vi "MuxReset.vi"(8 "error in (no error)":errorcluster, 11 "GPIBSwitching in":refnum<class "GPIBSwitching.lvclass">) -> (0 "error out":errorcluster, 3 "GPIBSwitching out":refnum<class "GPIBSwitching.lvclass">)   [LabVIEW 2018, in "GPIBSwitching.lvclass"]
uses:
  GPIBSwitching.lvclass
  C:/ProbeTestSoftware2019/itk-strip-sensor-qc/InstrControl/InstrControl.lvclass
  MUX_CommandsGlobal.vi
  InstrControl.lvclass
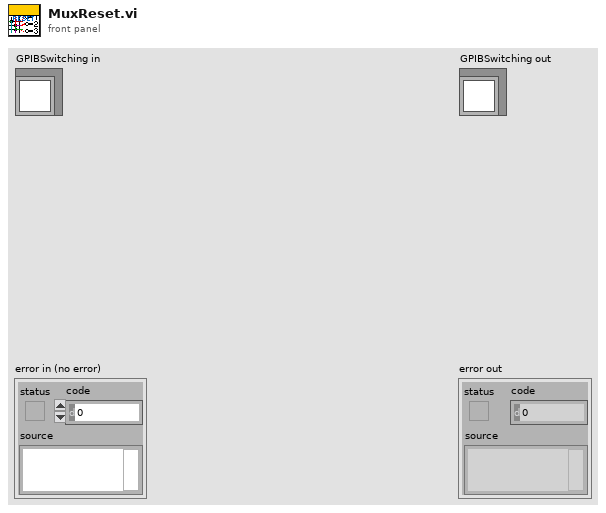
[diagram p1: front panel]
types:
  T1 = cluster{"Mux1 address":string, "Mux2 address":string, "Instrument name":string, "Instrument type":u16, "Command \"MUX Reset\"":string, "Command \"Select MUX Channel\"":string}
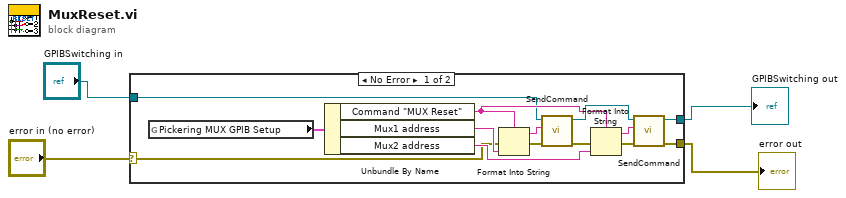
[diagram p0: block diagram]
diagram:
  n1 = case shown="No Error" "error in (no error)" {
    selector: "error in (no error)" -> [w5 w20]
    tunnel: [w13 w20] -> w3
    tunnel: [w17 w19] -> w4
    tunnel: "GPIBSwitching in" -> [w6 w19]
    frame No Error {
      n2 = global read "MUX_CommandsGlobal.vi" "Pickering MUX GPIB Setup"() -> (w12:T1)
      n3 = Unbundle By Name(w12) -> ("Command \"MUX Reset\""=w11:string, "Mux1 address"=w10:string, "Mux2 address"=w9:string)
      n4 = Format Into String(format string=w11, error in=w5, w10) -> (resulting string=w8:string, error out=w16:errorcluster)  [unwired: 1 in]
      n5 = call "SendCommand.vi"("error in (no error)"=w16, "Command string"=w8, "InstControl in"=w6) -> ("error out"=w15:errorcluster, "InstControl out"=w18:refnum<class "GPIBSwitching.lvclass">)  [unwired: 7 in]
      n6 = Format Into String(format string=w11, error in=w15, w9) -> (resulting string=w7:string, error out=w14:errorcluster)  [unwired: 1 in]
      n7 = call "SendCommand.vi"("error in (no error)"=w14, "Command string"=w7, "InstControl in"=w18) -> ("error out"=w13:errorcluster, "InstControl out"=w17:refnum<class "GPIBSwitching.lvclass">)  [unwired: 7 in]
    }
    frame Error {
    }
  }
  "error out" <- w3
  "GPIBSwitching out" <- w4
